vi "visa_resource_name_required.vi"(8 "error in (no error)":errorcluster, 11 "VI Ref":refnum<vi>) -> (0 "error out":errorcluster, 3 "VI Ref Out":refnum<vi>)   [LabVIEW 2018]
doc: "This test checks whether VISA Resource Name is a Required input on the connector pane. If the \"automatically correct the error\" is checked, it will automatically fix the error and save the vi to replace the original one."
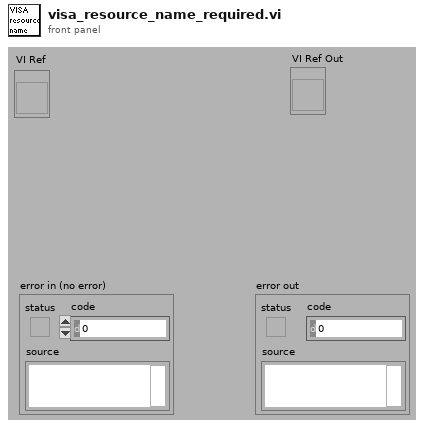
[diagram p1: front panel]
types:
  T1 = enum16{"Invalid Wire Rule", "Required", "Recommended", "Optional", "Dynamic Dispatch"}
  T2 = enum16{"Invalid Wire Rule", "Required", "Recommended", "Optional", "Dynamic Dispatch"}[]
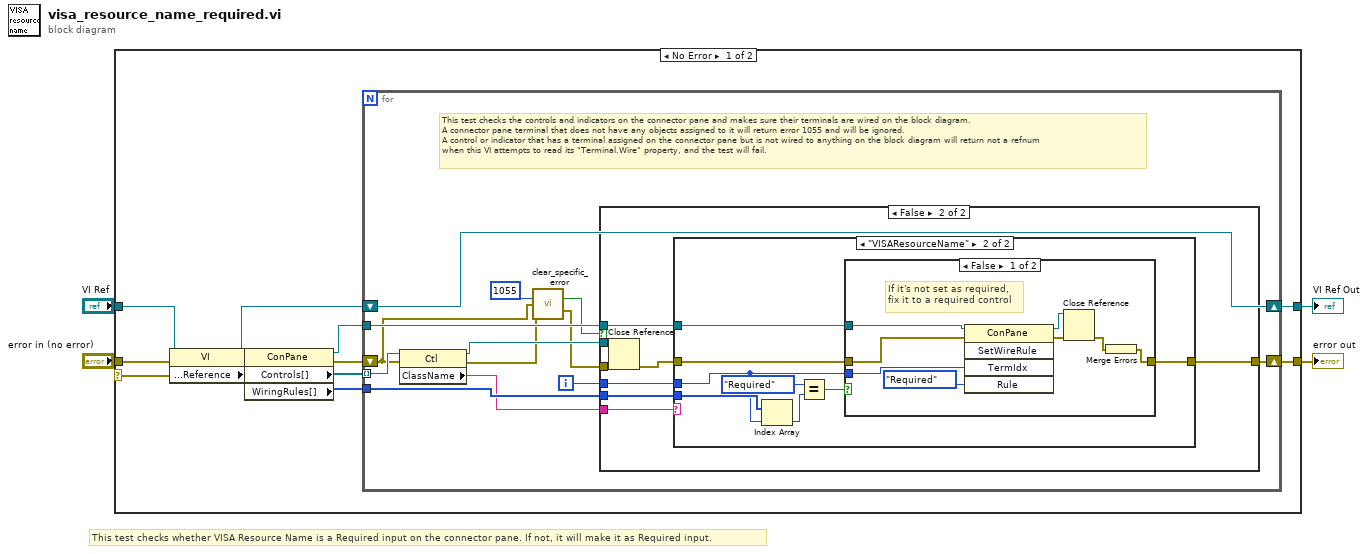
[diagram p0: block diagram]
diagram:
  # "This test checks whether VISA Resource Name is a Required input on the connector pane. If not, it will make it as Required input."
  n1 = case shown="No Error" "error in (no error)" {
    selector: "error in (no error)" -> [_ w57]
    tunnel: "VI Ref" -> [w15 w56]
    tunnel: [w10 w57] -> w3
    tunnel: [w9 w56] -> w2
    tunnel: "error in (no error)" -> [w8 _]
    frame No Error {
      n2 = property class="VI"(reference=w15, error in=w8) -> (reference out=w11:refnum<vi>, error out=w7:errorcluster, "Connector Pane:Reference"=w13:refnum<vi>)
      n3 = property class="ConPane"(reference=w13, error in=w7) -> (reference out=w6:refnum<vi>, error out=w5:errorcluster, "Controls[]"=w14:refnum<vi>[], "WiringRules[]"=w12:T2)
      n4 = for {
        tunnel: w14 -> [w25] mode=indexing
        shift-right: [w22] -> w10
        shift-left: w5 -> [w19]
        tunnel: w12 -> [w27]
        tunnel: w6 -> [w26]
        shift-right: [w21] -> w9
        shift-left: w11 -> [w21]
        i -> [w28]
        # "This test checks the controls and indicators on the connector pane and makes sure their terminals are wired on the block diagram.\nA connector pane terminal that does not have any objects assigned to it will return error 1055 and will be ignored.\nA control or indicator that has a terminal assigned on the connector pane but is not wired to anything on the block diagram will return not a refnum \nwhen this VI attempts to read its \"Terminal.Wire\" property, and the test will fail."
        n5 = property class="Ctl"(reference=w25, error in=w19) -> (reference out=w23:refnum<vi>, error out=w18:errorcluster, "ClassName"=w24:string)
        n6 = call "clear_specific_error.vi"("Error of Interest"=1055, "error in (previous)"=w19, "error in (current)"=w18) -> ("Specific Error?"=w16:bool, "error out"=w17:errorcluster)  [unwired: 11 out]
        n7 = case shown="False" w16 {
          tunnel: w28 -> [_ w37]
          tunnel: w27 -> [_ w36]
          tunnel: w26 -> [_ w35]
          tunnel: w24 -> [_ w34]
          tunnel: w23 -> [_ w33]
          tunnel: [w29 w32] -> w22
          tunnel: w17 -> [w29 w31]
          frame True {
          }
          frame False {
            n8 = Close Reference(reference=w33, error in (no error)=w31) -> (error out=w30:errorcluster)
            n9 = case shown="\"VISAResourceName\"" w34 {
              tunnel: w37 -> [_ w41]
              tunnel: w36 -> [_ w46]
              tunnel: w35 -> [_ w42]
              tunnel: w30 -> [w38 w40]
              tunnel: [w38 w39] -> w32
              frame Default {
              }
              frame "VISAResourceName" {
                n10 = Index Array(array=w46, index=w41) -> (element=w44:T1)
                n11 = Equal?(x=T1."Required" ("Wire Rule"), y=w44) -> (x = y?=w43:bool)
                n12 = case shown="False" w43 {
                  tunnel: w42 -> [w54 _]
                  tunnel: w41 -> [w52 _]
                  tunnel: w40 -> [w51 w55]
                  tunnel: [w50 w55] -> w39
                  frame False {
                    # "If it's not set as required,\nfix it to a required control"
                    n13 = invoke class="ConPane" method="SetWireRule"(reference=w54, error in=w51, "TermIdx"=w52, "Rule"=T1."Required") -> (reference out=w49:refnum<vi>, error out=w48:errorcluster)  [unwired: 1 in, 3 out]
                    n14 = Close Reference(reference=w49, error in (no error)=w48) -> (error out=w47:errorcluster)
                    n15 = Merge Errors(w47) -> (w50:errorcluster)
                  }
                  frame True {
                  }
                }
              }
            }
          }
        }
      }
    }
    frame Error {
    }
  }
  "error out" <- w3
  "VI Ref Out" <- w2
